vi "Core Execute.vi"(8 "error in (no error)":errorcluster, 11 "CIFTemplateNode in":refnum<class "CIFCorePlugin.lvclass">) -> (0 "error out":errorcluster, 3 "CIFTemplateNode out":refnum<class "CIFCorePlugin.lvclass">)   [LabVIEW 2021, in "CIFCorePlugin.lvclass"]
uses:
  CIFCorePlugin.lvclass
  CIFCorePlugin.lvclass/CIFCorePlugin.ctl
  Typedef/Energized States.ctl
  <vilib>/CIF Foundation/CIF Utilities/Time/System Time/Get System Time.vi
  Accessors/Timestamps/Write Execute TS.vi
  <vilib>/Utility/error.llb/Clear Errors.vi
  <vilib>/CIF Foundation/CIF Utilities/Time/System Time/Sleep Until Future Time.vi
  Accessors/Read Sleep Limits (ns).vi
  Accessors/Timestamps/Write Target Wake TS.vi
  SubVIs/Start Running.vi
  Common/Utilities/Add Error.vi
  Accessors/Read Plugin Name.vi
  Accessors/Timestamps/Read Running TS.vi
  Accessors/Read Running Internal Data.vi
  Accessors/Read Timing Override.vi
  Accessors/Read Common Config.vi
  <vilib>/CIF Foundation/CIF Utilities/Time/System Time/LabVIEW Time to TAI Time.vi
  <vilib>/CIF Foundation/CIF Utilities/Time/SubVIs/Add Error.vi
  <vilib>/CIF Foundation/CIF Utilities/Errors/Append Error Location.vi
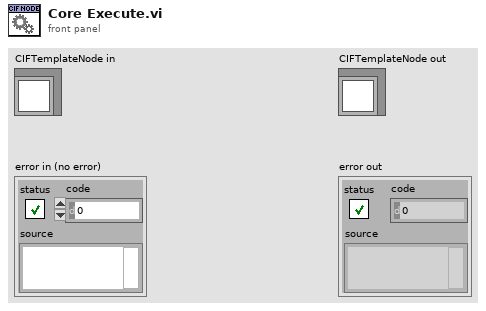
[diagram p1: front panel]
types:
  T1 = typedef "CIFCorePlugin.lvclass/Energized States.ctl" = enum16{"Listen", "Prepare", "Execute", "Housekeep", "Cleanup", "Destroy"}
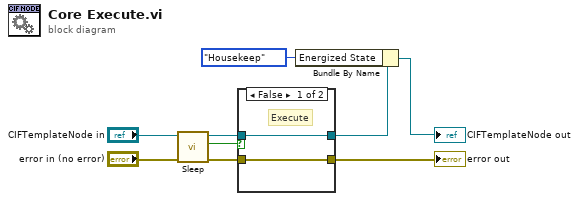
[diagram p0: block diagram]
diagram:
  n1 = call "Sleep.vi"("error in (no error)"="error in (no error)", "CIFCorePlugin in"="CIFTemplateNode in") -> ("error out"=w4:errorcluster, "Housekeep only"=w3:bool, "CIFCorePlugin out"=w5:refnum<class "CIFCorePlugin.lvclass">)  [unwired: 7 in]
  n2 = case shown="False" w3 {
    tunnel: [w11 w12] -> w9
    tunnel: [w10 w13] -> w7
    tunnel: w5 -> [w10 w13]
    tunnel: w4 -> [w11 w12]
    frame False {
      # "Execute"
    }
    frame True {
    }
  }
  "error out" <- w9
  n3 = Bundle By Name(cluster=w7, "Energized State"=Energized_States."Housekeep") -> (→"CIFTemplateNode out":refnum<class "CIFCorePlugin.lvclass">)
